vi "FTIR_1.vi"() -> ()   [LabVIEW 2021]
uses:
  <vilib>/express/express analysis/Spectral/Block/exnSpectralBlock spectral measurements power poly.vi
  <vilib>/express/express analysis/Spectral/Block/exnSpectralBlock spectral measurements power WFM.vi
  <vilib>/express/express analysis/Spectral/XNode/ExpressSpectralMeasurementsBlockNode.xnode
panel:
  out "Waveform Graph":cluster{"f0":dbl, "df":dbl, "magnitude":dbl[]}(graph)
  out "Waveform signal 2":cluster{"time":dbl[], dbl[]}(graph)
  out "time":dbl[](array[numeric])
  in  "Mirror 1 distance (m)":dbl
  out "Wavenumber k":dbl
  out "Mirror 2 frequency (Hz)":dbl
  out "Mirror 1 frequency (Hz)":dbl
  out "Phase (deg.)":dbl
  in  "Mirror speed (m/s)":dbl(slide) scale=0.0..100.0
  in  "Wavelength (m)":dbl(slide) scale=0.0..1.0
  out "Waveform signal":cluster{"time":dbl[], dbl[]}(graph)
  in  "no. of samples":dbl
  in  "end time":dbl
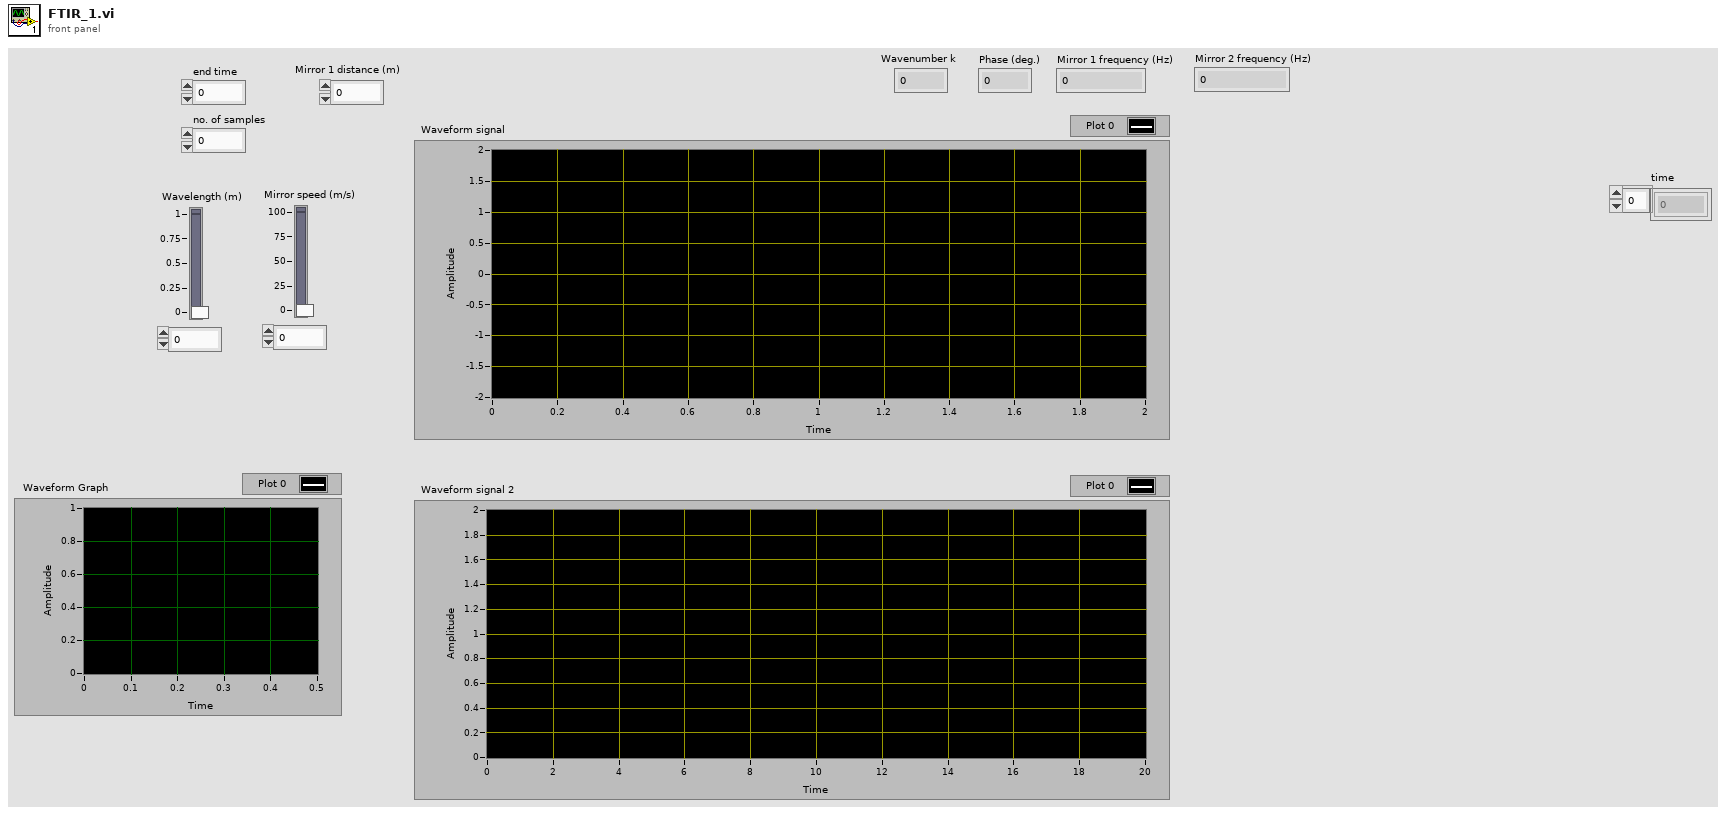
[diagram p1: front panel]
types:
  T1 = cluster{"averaging mode":u16, "weighting mode":u16, "number of averages":u32}
  T2 = cluster{"dB On (F)":bool, "unwrap phase (F)":bool, "convert to degree (F)":bool}
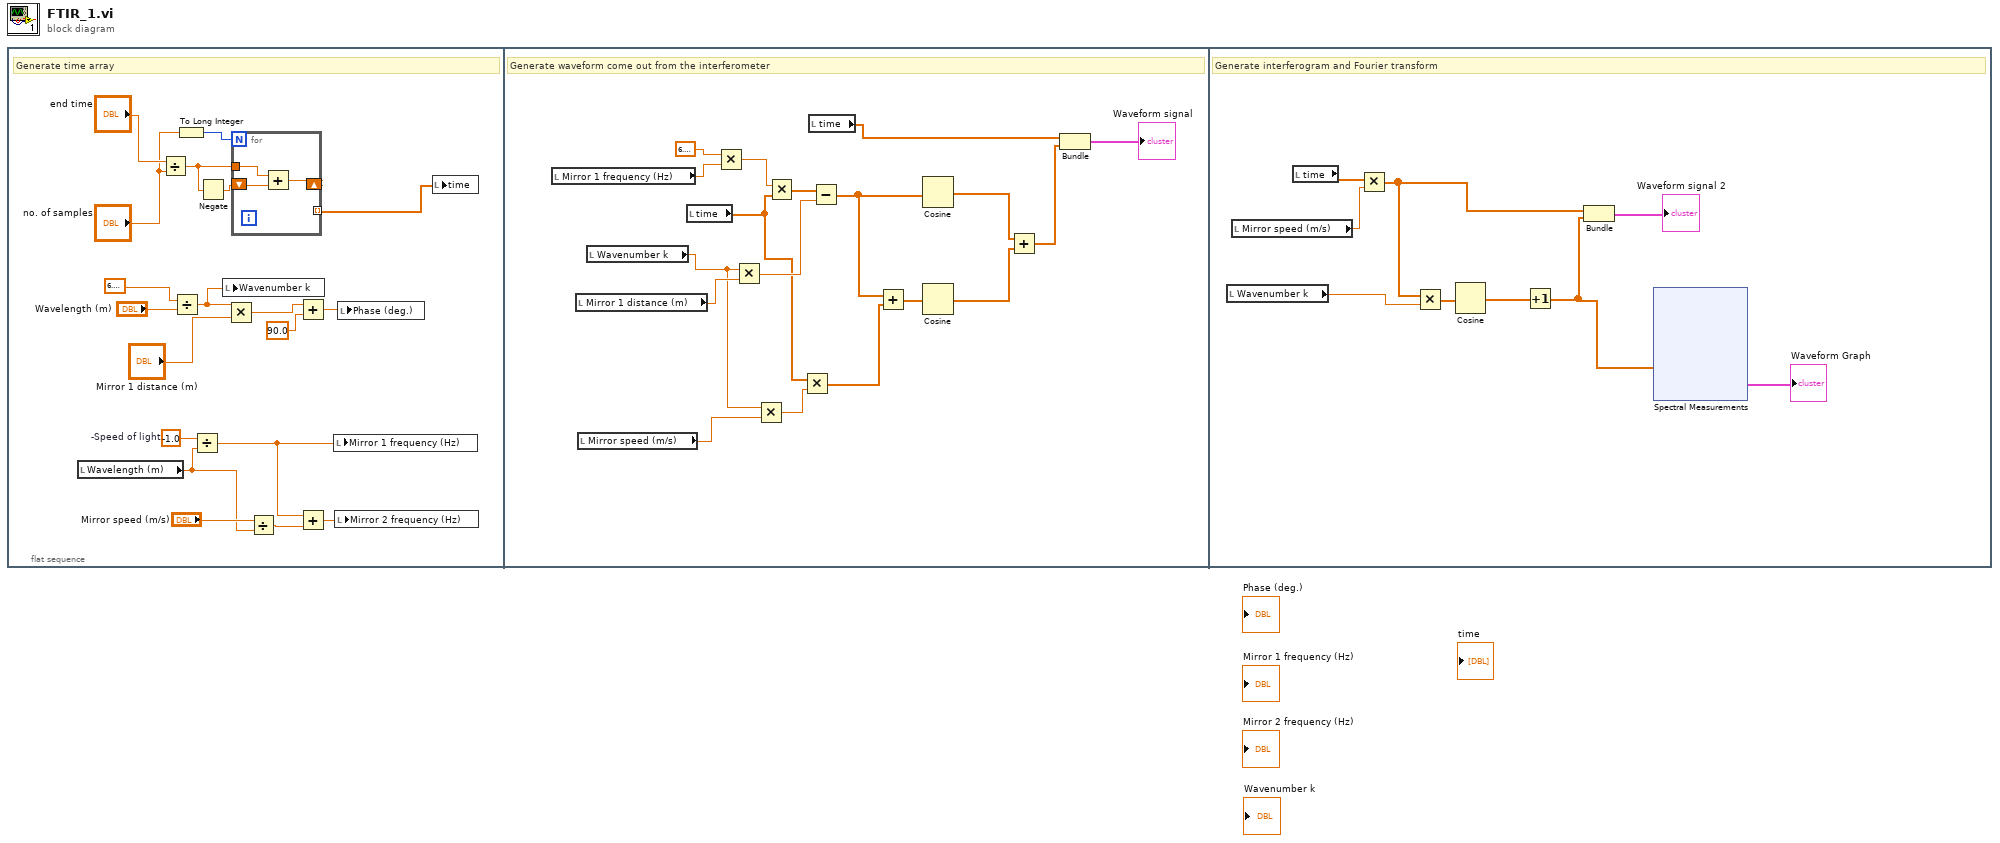
[diagram p0: block diagram]
diagram:
  n1 = flat-sequence {
    frame #0 {
      w10 = -1.0  # -Speed of light
      # "Generate time array"
      n2 = local read "Wavelength (m)"() -> (w8:dbl)
      n3 = Divide(x="end time", y="no. of samples") -> (x/y=w18:dbl)
      n4 = Divide(x=6.283185307179586, y="Wavelength (m)") -> (x/y=w5:dbl)
      n5 = To Long Integer(number="no. of samples") -> (32bit integer=w19:i32)
      n6 = Divide(x=w10, y=w8) -> (x/y=w2:dbl)
      n7 = Negate(x=w18) -> (-x=w17:dbl)
      n8 = local write "Wavenumber k"(w5) -> ()
      n9 = Multiply(x=w5, y="Mirror 1 distance (m)") -> (x*y=w4:dbl)
      n10 = for {
        N: w19 -> [_]
        shift-right: [w20] -> _
        shift-left: w17 -> [w21]
        tunnel: w18 -> [w22]
        tunnel: [w20] -> w14 mode=indexing
        n11 = Add(x=w22, y=w21) -> (x+y=w20:dbl)
      }
      n12 = Divide(x="Mirror speed (m/s)", y=w8) -> (x/y=w1:dbl)
      n13 = Add(x=w4, y=90.0) -> (x+y=w11:dbl)
      n14 = Add(x=w2, y=w1) -> (x+y=w7:dbl)
      n15 = local write "Mirror 1 frequency (Hz)"(w2) -> ()
      n16 = local write "Mirror 2 frequency (Hz)"(w7) -> ()
      n17 = local write "Phase (deg.)"(w11) -> ()
      n18 = local write "time"(w14) -> ()
    }
    frame #1 {
      # "Generate waveform come out from the interferometer"
      n19 = local read "Mirror 1 frequency (Hz)"() -> (w40:dbl)
      n20 = local read "Mirror 1 distance (m)"() -> (w36:dbl)
      n21 = local read "Mirror speed (m/s)"() -> (w32:dbl)
      n22 = local read "Wavenumber k"() -> (w29:dbl)
      n23 = local read "time"() -> (w30:dbl[])
      n24 = Multiply(x=6.283185307179586, y=w40) -> (x*y=w38:dbl)
      n25 = Multiply(x=w29, y=w36) -> (x*y=w35:dbl)
      n26 = Multiply(x=w29, y=w32) -> (x*y=w31:dbl)
      n27 = Multiply(x=w38, y=w30) -> (x*y=w37:dbl[])
      n28 = Multiply(x=w30, y=w31) -> (x*y=w28:dbl[])
      n29 = local read "time"() -> (w25:dbl[])
      n30 = Subtract(x=w37, y=w35) -> (x-y=w33:dbl[])
      n31 = Add(x=w33, y=w28) -> (x+y=w34:dbl[])
      n32 = Cosine(x=w33) -> (cos(x)=w27:dbl[])
      n33 = Cosine(x=w34) -> (cos(x)=w26:dbl[])
      n34 = Add(x=w27, y=w26) -> (x+y=w24:dbl[])
      n35 = Bundle("time"=w25, w24) -> (→"Waveform signal":cluster{"time":dbl[], dbl[]})  [unwired: 1 in]
    }
    frame #2 {
      # "Generate interferogram and Fourier transform"
      n36 = local read "Wavenumber k"() -> (w45:dbl)
      n37 = local read "Mirror speed (m/s)"() -> (w47:dbl)
      n38 = local read "time"() -> (w48:dbl[])
      n39 = Multiply(x=w48, y=w47) -> (x*y=w43:dbl[])
      n40 = Multiply(x=w43, y=w45) -> (x*y=w44:dbl[])
      n41 = Cosine(x=w44) -> (cos(x)=w46:dbl[])
      n42 = Increment(x=w46) -> (x+1=w42:dbl[])
      n43 = Bundle(w43, w42) -> (→"Waveform signal 2":cluster{dbl[], dbl[]})  [unwired: 1 in]
      n44 = xnode "Spectral Measurements"("Signals"=w42) -> ("Power Spectrum"=→"Waveform Graph":cluster{"f0":dbl, "df":dbl, "magnitude":dbl[]})  [unwired: 1 in, 1 out]
    }
  }
